vi "deleave.vi"(11 "Data":u64[](array[numeric])) -> (2 "Counts":i16[][](array[numeric]), 3 "Voltage":dbl[][](array[numeric]))   [LabVIEW 2014]
doc: "Deleave and convert Data. Deleaves data from DMA readout and converts with SubVIs to counts and voltages."
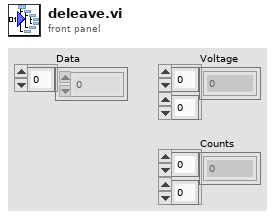
[diagram p1: front panel]
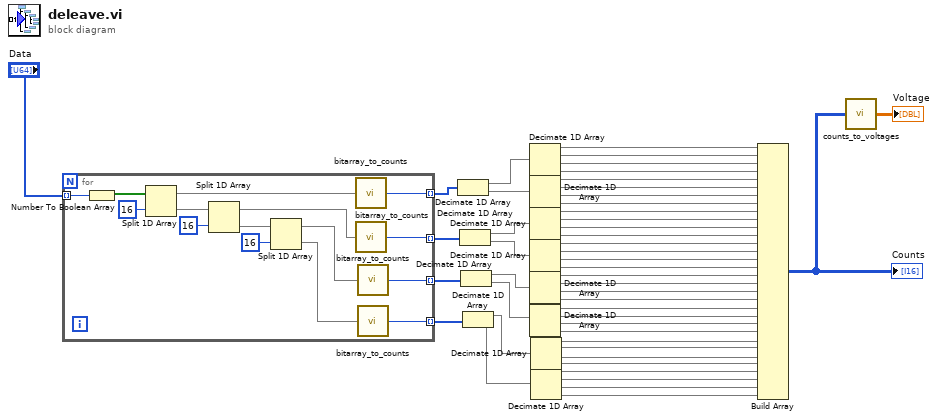
[diagram p0: block diagram]
diagram:
  n1 = for {
    tunnel: "Data" -> [w62] mode=indexing
    tunnel: [w54] -> w2 mode=indexing
    tunnel: [w52] -> w3 mode=indexing
    tunnel: [w50] -> w4 mode=indexing
    tunnel: [w49] -> w5 mode=indexing
    n2 = Number To Boolean Array(number=w62) -> (Boolean array=w61:bool[])
    n3 = Split 1D Array(array=w61, index=16) -> (first subarray=w55:bool[], second subarray=w59:bool[])
    n4 = Split 1D Array(array=w59, index=16) -> (first subarray=w53:bool[], second subarray=w56:bool[])
    n5 = Split 1D Array(array=w56, index=16) -> (first subarray=w51:bool[], second subarray=w48:bool[])
    n6 = call "bitarray_to_counts.vi"("16Bit Array"=w55) -> ("Counts"=w54:i16)
    n7 = call "bitarray_to_counts.vi"("16Bit Array"=w53) -> ("Counts"=w52:i16)
    n8 = call "bitarray_to_counts.vi"("16Bit Array"=w51) -> ("Counts"=w50:i16)
    n9 = call "bitarray_to_counts.vi"("16Bit Array"=w48) -> ("Counts"=w49:i16)
  }
  n10 = Decimate 1D Array(w2) -> (w6:i16[], w7:i16[])
  n11 = Decimate 1D Array(w3) -> (w9:i16[], w8:i16[])
  n12 = Decimate 1D Array(w4) -> (w10:i16[], w11:i16[])
  n13 = Decimate 1D Array(w5) -> (w12:i16[], w13:i16[])
  n14 = Decimate 1D Array(w6) -> (w14:i16[], w15:i16[], w16:i16[], w17:i16[])
  n15 = Decimate 1D Array(w7) -> (w18:i16[], w19:i16[], w20:i16[], w21:i16[])
  n16 = Decimate 1D Array(w9) -> (w22:i16[], w23:i16[], w24:i16[], w25:i16[])
  n17 = Decimate 1D Array(w8) -> (w26:i16[], w27:i16[], w28:i16[], w29:i16[])
  n18 = Decimate 1D Array(w10) -> (w30:i16[], w31:i16[], w32:i16[], w33:i16[])
  n19 = Decimate 1D Array(w11) -> (w34:i16[], w35:i16[], w36:i16[], w37:i16[])
  n20 = Decimate 1D Array(w12) -> (w38:i16[], w39:i16[], w40:i16[], w41:i16[])
  n21 = Decimate 1D Array(w13) -> (w42:i16[], w43:i16[], w44:i16[], w45:i16[])
  n22 = Build Array(w14, w15, w16, w17, w18, w19, w20, w21, w22, w23, w24, w25, w26, w27, w28, w29, w30, w31, w32, w33, w34, w35, w36, w37, w38, w39, w40, w41, w42, w43, w44, w45) -> (w46:i16[][])
  "Counts" <- w46
  n23 = call "counts_to_voltages.vi"("Count Array"=w46) -> ("Voltage Array"=→"Voltage":dbl[][])
